vi "Read.vi"(6 "Close (F)":bool, 8 "error in (no error)":errorcluster, 9 "timeout in ms (-1)":i32=-1, 10 "ignore previous (F)":bool, 11 "Tag in":refnum<class "Tag.lvclass">) -> (0 "error out":errorcluster, 1 "timed out?":bool, 2 "Element":T1, 3 "Tag out":refnum<class "Tag.lvclass">, 4 "New Value?":bool, 5 "Time Stamp":timestamp, 7 "Sequence":u64)   [LabVIEW 2022 SP3, in "Enclave.lvlib" / "Tag.lvclass"]
uses:
  Tag.lvclass
  Element.ctl
  Tag.lvclass/Tag.ctl
  Enclave.lvlib
  Enclave/Enclave.lvclass
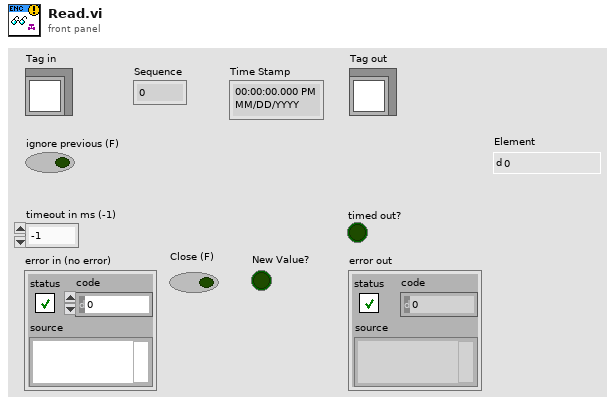
[diagram p1: front panel]
types:
  T1 = typedef "Enclave.lvlib/Element.ctl" = dbl
  T2 = typedef "Enclave.lvlib/Tag Data.ctl" = cluster{"Element":T1, "Sequence":u64, "Time Stamp":timestamp}
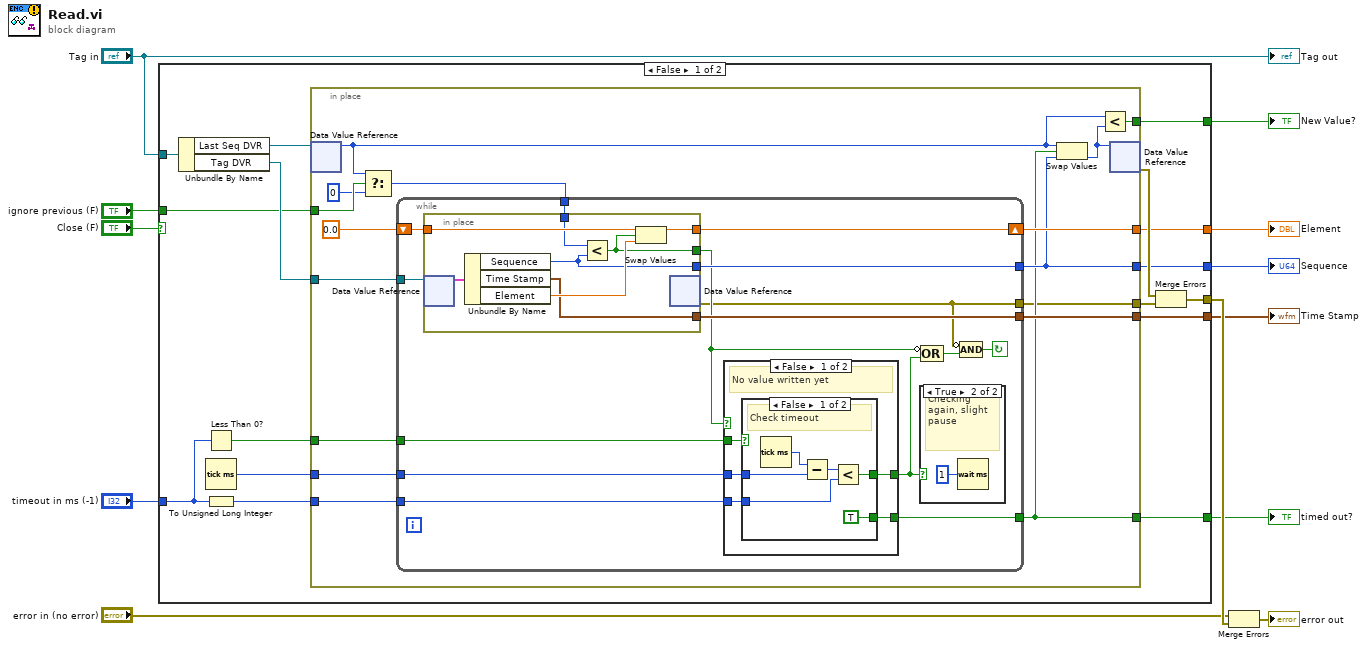
[diagram p0: block diagram]
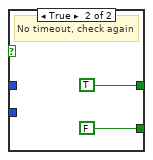
[diagram p2: hidden frame]
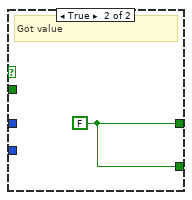
[diagram p3: hidden frame]
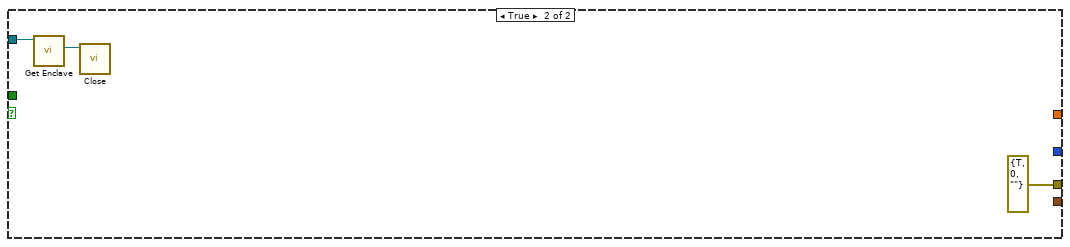
[diagram p5: hidden frame]
diagram:
  n1 = case shown="False" "Close (F)" {
    tunnel: "Tag in" -> [w26 w85]
    tunnel: [w24 _] -> w10
    tunnel: [w23 _] -> w9
    tunnel: [w22 _] -> w8
    tunnel: [w21 _] -> w7
    tunnel: [w18 _] -> w6
    tunnel: "timeout in ms (-1)" -> [w16 _]
    tunnel: "ignore previous (F)" -> [w14 _]
    tunnel: [w13 errorcluster {"status"=TRUE, "code"=0, "source"=""} ("error IO")] -> w12
    frame False {
      n2 = Unbundle By Name(w26) -> ("Last Seq DVR"=w17:refnum<data-value>, "Tag DVR"=w25:refnum<data-value>)
      n3 = Less Than 0?(x=w16) -> (x < 0?=w15:bool)
      n4 = Tick Count (ms)() -> (millisecond timer value=w20:u32)
      n5 = To Unsigned Long Integer(number=w16) -> (unsigned 32bit integer=w19:u32)
      n6 = in-place {
        in-place-border: w25 -> [w44]
        in-place-border: [w42] -> w24
        in-place-border: [w41] -> w23
        in-place-border: [w37] -> w22
        in-place-border: [w38] -> w21
        in-place-border: w20 -> [w40]
        in-place-border: w19 -> [w39]
        in-place-border: [w35] -> w18
        in-place-border: w15 -> [w34]
        in-place-border: w14 -> [w32]
        in-place-border: [w29] -> w27
        n7 = in-place-dvr #1(w17) -> (w33:u64)  [unwired: 1 out]
        n8 = Select(t=w33, s=w32, f=u64 0 ("t")) -> (s? t:f=w30:u64)
        n9 = while {
          tunnel: w44 -> [w59]
          shift-right: [w57] -> w42
          shift-left: T1 0.0 ("Element") -> [w58]
          tunnel: [w56] -> w41
          tunnel: [w54] -> w37
          tunnel: [w55] -> w38
          tunnel: w40 -> [w53]
          tunnel: w39 -> [w52]
          tunnel: w34 -> [w50]
          tunnel: w30 -> [w49]
          tunnel: [w45] -> w29
          stop <- w46 continue-if-true
          n10 = in-place {
            in-place-border: w58 -> [w80]
            in-place-border: [w78] -> w57
            in-place-border: [w77] -> w56
            in-place-border: [w76] -> w51
            in-place-border: [w75] -> w55
            in-place-border: w49 -> [w74]
            n11 = in-place-dvr #2(w59) -> (w81:T2)  [unwired: 1 out]
            n12 = Unbundle By Name(w81) -> ("Sequence"=w75:u64, "Time Stamp"=w77:timestamp, "Element"=w79:T1)
            n13 = Less?(x=w74, y=w75) -> (x < y?=w76:bool)
            n14 = Swap Values(12:w80, 13:w76, 14:w79) -> (1:w78:T1)  [unwired: 1 out]
            n15 = in-place-dvr #2() -> (w45:errorcluster)  [unwired: 1 in, 1 out]
          }
          n16 = case shown="False" w51 {
            tunnel: w53 -> [w64 _]
            tunnel: w52 -> [w63 _]
            tunnel: [w62 w73] -> w54
            tunnel: w50 -> [w61 _]
            tunnel: [w60 w73] -> w48
            frame False {
              # "No value written yet"
              n17 = case shown="False" w61 {
                tunnel: w64 -> [w70 _]
                tunnel: w63 -> [w67 _]
                tunnel: [TRUE FALSE] -> w62
                tunnel: [w65 TRUE] -> w60
                frame False {
                  # "Check timeout"
                  n18 = Tick Count (ms)() -> (millisecond timer value=w69:u32)
                  n19 = Subtract(x=w69, y=w70) -> (x-y=w68:u32)
                  n20 = Less?(x=w68, y=w67) -> (x < y?=w65:bool)
                }
                frame True {
                  # "No timeout, check again"
                }
              }
            }
            frame True {
              w73 = FALSE
              # "Got value"
            }
          }
          n21 = case shown="True" w48 {
            frame False {
            }
            frame True {
              # "Checking again, slight pause"
              n22 = Wait (ms)(milliseconds to wait=u32 1) -> ()  [unwired: 1 out]
            }
          }
          n23 = Compound Arithmetic op=OR(invert w51, w48) -> (w47:bool)
          n24 = Compound Arithmetic op=AND(invert w45, w47) -> (w46:bool)
        }
        n25 = Swap Values(12:w33, 13:w37, 14:w38) -> (3:w36:u64)  [unwired: 1 out]
        n26 = Less?(x=w33, y=w36) -> (x < y?=w35:bool)
        n27 = in-place-dvr #1(w36) -> (w28:errorcluster)  [unwired: 1 out]
      }
      n28 = Merge Errors(w28, w27) -> (w13:errorcluster)
    }
    frame True {
      n29 = call "Get Enclave.vi"("Tag in"=w85) -> ("Enclave"=w84:refnum<class "Enclave.lvclass">)  [unwired: 8 in, 2 out]
      n30 = call "Close.vi"("Enclave in"=w84) -> ()  [unwired: 10 in, 1 out]
    }
  }
  "timed out?" <- w8
  "Element" <- w10
  "Time Stamp" <- w9
  "Sequence" <- w7
  "New Value?" <- w6
  n31 = Merge Errors("error in (no error)", w12) -> (→"error out":errorcluster)
  "Tag out" <- "Tag in"
